vi "ep_Load Speed Torque.vi"(8 "error in (no error)":errorcluster, 10 "speed [RPM]":dbl, 11 "load [W]":dbl) -> (0 "error out":errorcluster, 3 "torque [Nm]":dbl)   [LabVIEW 2014, in "NI_EP_Motor Monitoring.lvlib"]
uses:
  <vilib>/addons/Electrical Power/Motor Monitoring/NI_EP_Motor Monitoring.lvlib
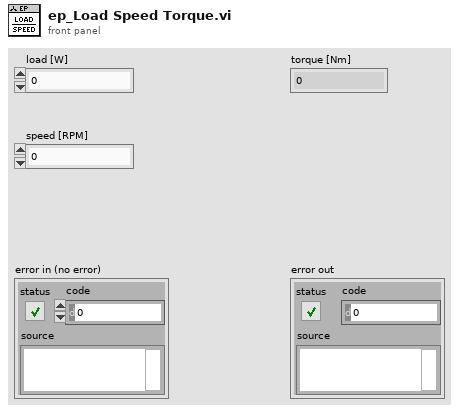
[diagram p1: front panel]
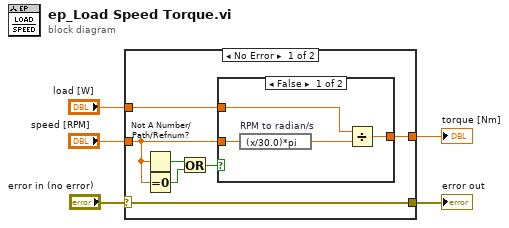
[diagram p0: block diagram]
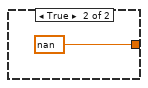
[diagram p2: hidden frame]
diagram:
  n1 = case shown="No Error" "error in (no error)" {
    selector: "error in (no error)" -> [w9 w18]
    tunnel: "speed [RPM]" -> [w6 _]
    tunnel: [w9 w18] -> w3
    tunnel: [w8 _] -> w2
    tunnel: "load [W]" -> [w7 _]
    frame No Error {
      n2 = Not A Number/Path/Refnum?(number/path/refnum=w6) -> (NaN/Path/Refnum?=w11:bool)
      n3 = Equal To 0?(x=w6) -> (x = 0?=w12:bool)
      n4 = Or(x=w11, y=w12) -> (x .or. y?=w10:bool)
      n5 = case shown="False" w10 {
        tunnel: [w13 nan] -> w8
        tunnel: w7 -> [w14 _]
        tunnel: w6 -> [w16 _]
        frame False {
          n6 = expression code="(x/30.0)*pi" "RPM to radian/s"(w16) -> (w15:dbl)
          n7 = Divide(x=w14, y=w15) -> (x/y=w13:dbl)
        }
        frame True {
        }
      }
    }
    frame Error {
    }
  }
  "error out" <- w3
  "torque [Nm]" <- w2
